vi "MesaurementTime.vi"() -> ()   [LabVIEW 2011]
panel:
  in  "Mesaurement line":dbl
  in  "Mesaurement stack":dbl
  in  "Mesaurement time area":dbl
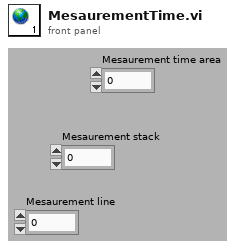
[diagram p1: front panel]
diagram:
